vi "Pick Up Order.vi"(8 "error in (no error)":errorcluster, 10 "Beverage.lvclass":refnum<class "Beverage.lvclass">, 11 "Customer in":refnum<class "Customer.lvclass">) -> (0 "error out":errorcluster, 3 "Customer out":refnum<class "Customer.lvclass">)   [LabVIEW 2020, in "Customer.lvclass"]
uses:
  Customer.lvclass
  Support/Beverages/Beverage/Beverage.lvclass
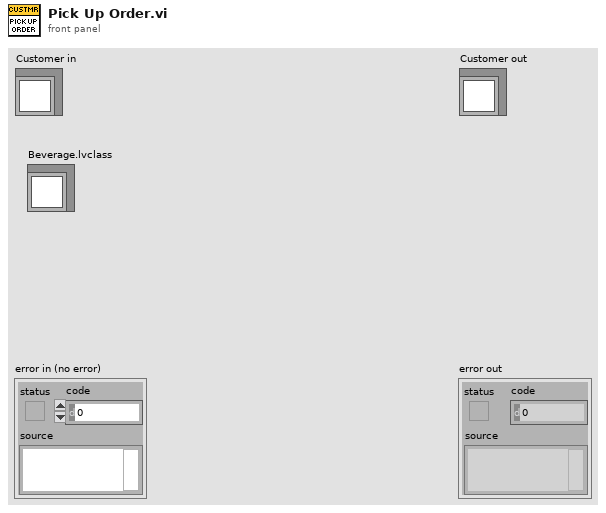
[diagram p1: front panel]
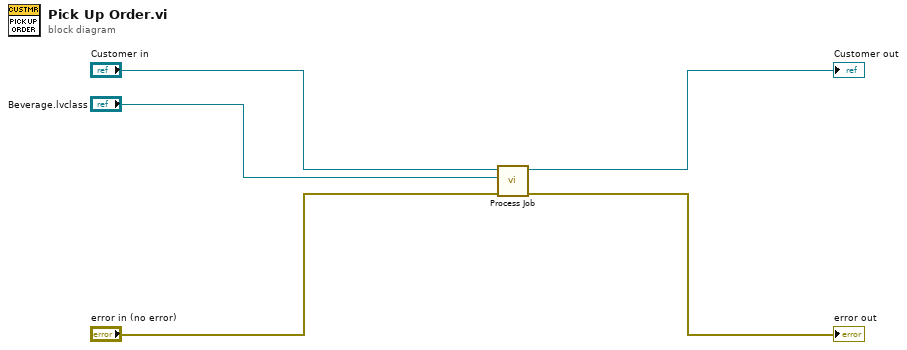
[diagram p0: block diagram]
diagram:
  n1 = call-dynamic "Process Job.vi"("error in (no error)"="error in (no error)", "Job"="Beverage.lvclass", "Process Job In"="Customer in") -> ("error out"=→"error out":errorcluster, "Process Job Out"=→"Customer out":refnum<class "Customer.lvclass">)  [unwired: 7 in]
